vi "Prep_Data_DAQ.vi"(8 "Error  in":errorcluster, 11 "Sequence":T2) -> (0 "Error out":errorcluster, 1 "Time Unit":T1(ring), 2 "Period (s )=Sample Numbers / Sample Frequency":dbl=5.0, 3 "Final Sending Data":u32[](array[numeric]), 4 "Sample Numbers":u32=20000000, 6 "Sample Frequency (Hz)":u32=1000000)   [LabVIEW 2021]
uses:
  DAQ_Control_1.ctl
  Global_DAQ.vi
  <vilib>/Utility/error.llb/Error Cluster From Error Code.vi
  <vilib>/ErrorRing/Error Ring.xnode
panel:
  out "Single line Data":u32[](array[numeric])
  out "Longest length":u32
  out "Array 2":u32[][](array[numeric])
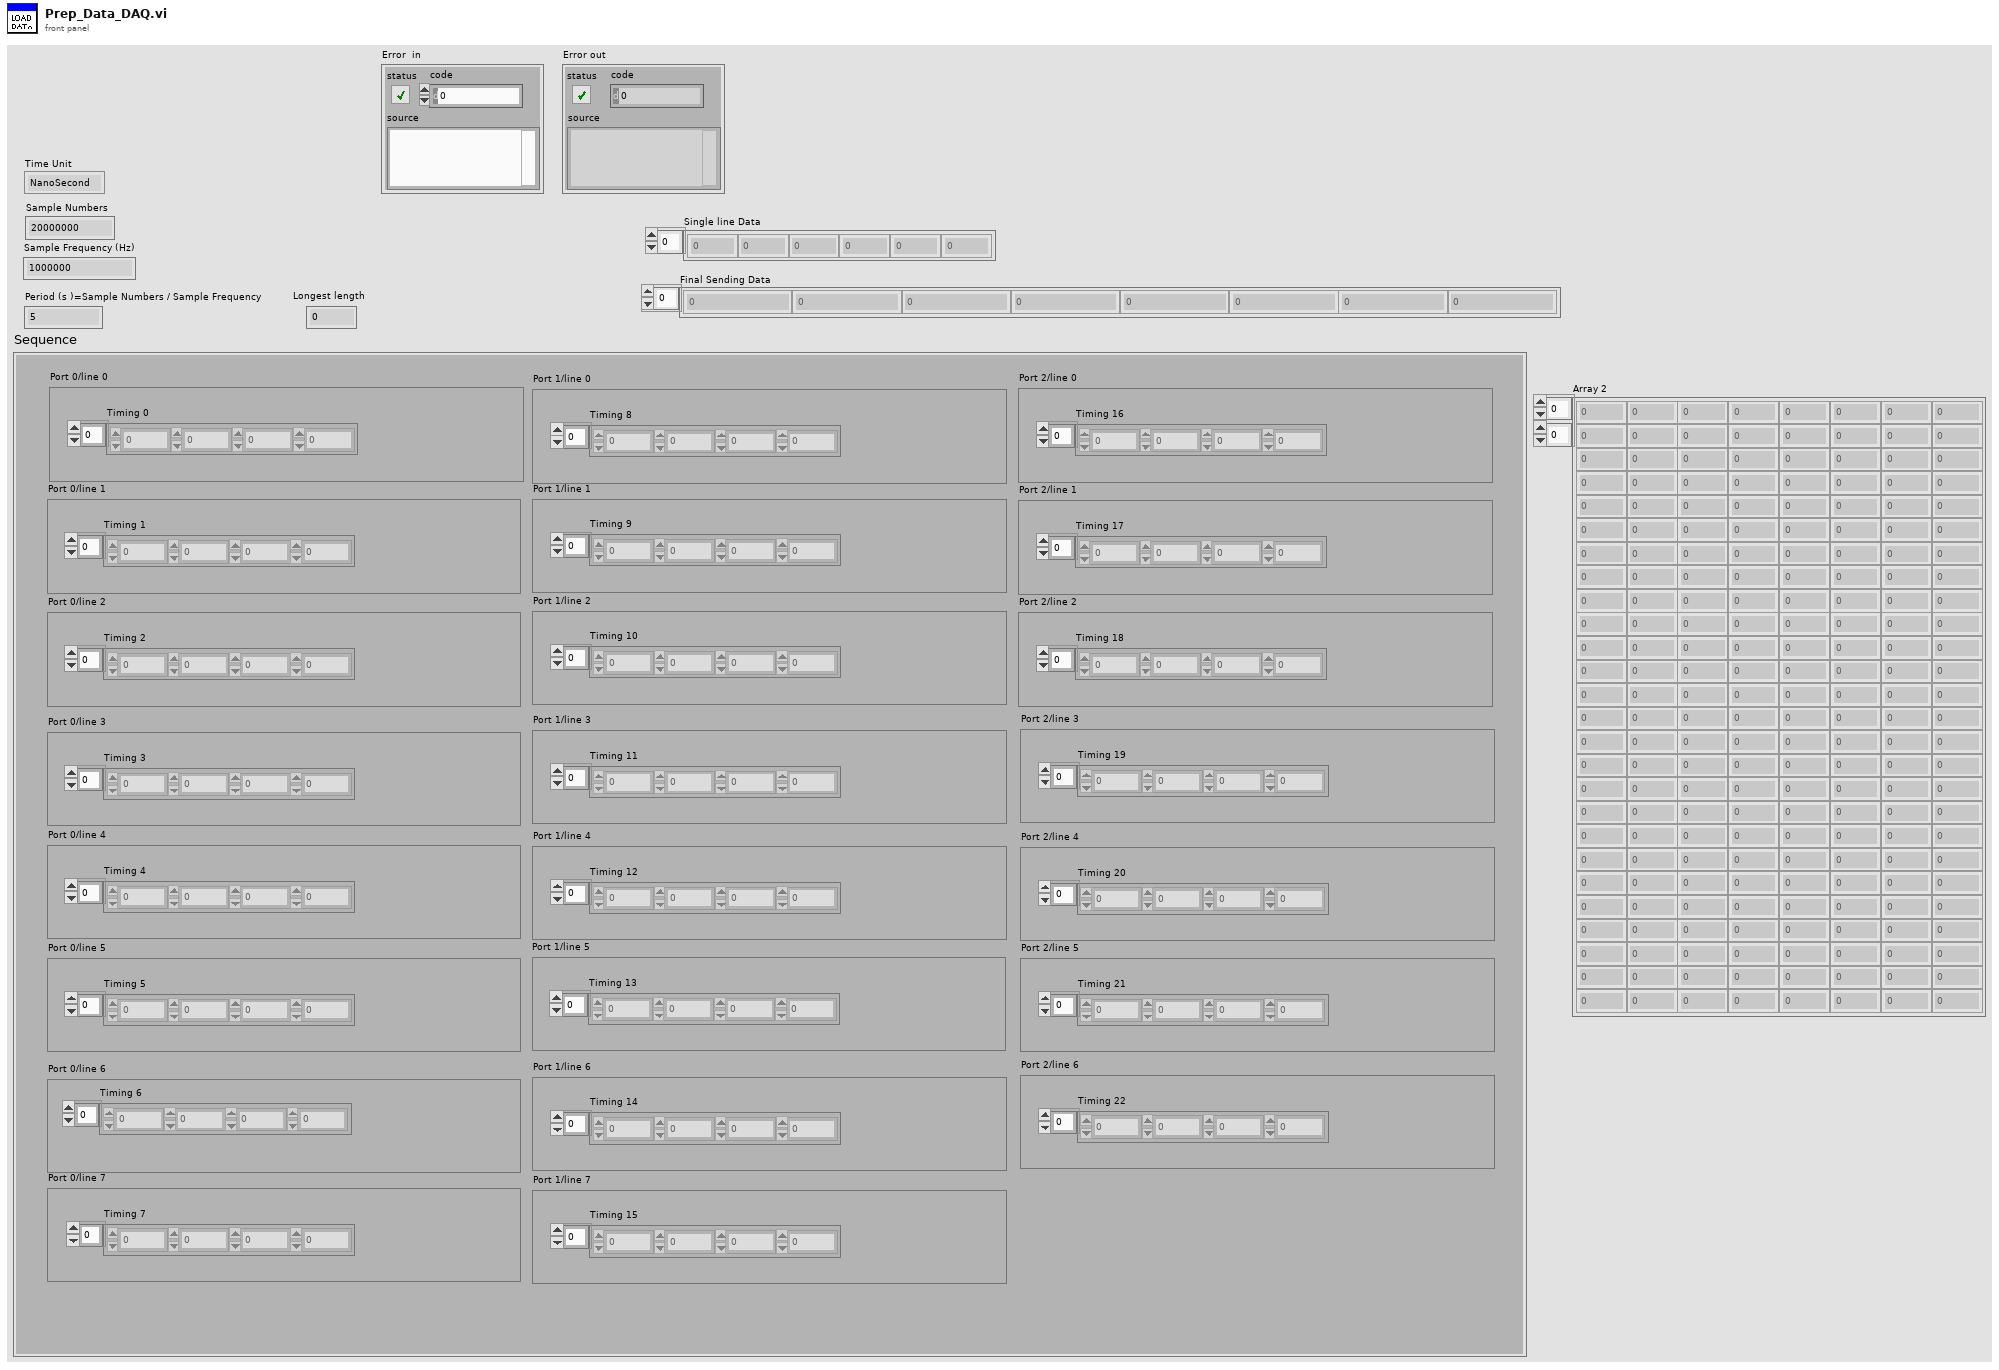
[diagram p1: front panel]
types:
  T1 = enum16{"NanoSecond", "MicroSecond", "MilliSecond"}
  T2 = typedef "DAQ_Control_1.ctl" = cluster{"Port 2/line 6":cluster{"Timing 22":dbl[]}, "Port 2/line 5":cluster{"Timing 21":dbl[]}, "Port 2/line 4":cluster{"Timing 20":dbl[]}, "Port 2/line 3":cluster{"Timing 19":dbl[]}, "Port 2/line 2":cluster{"Timing 18":dbl[]}, "Port 2/line 1":cluster{"Timing 17":dbl[]}, "Port 2/line 0":cluster{"Timing 16":dbl[]}, "Port 1/line 7":cluster{"Timing 15":dbl[]}, "Port 1/line 6":cluster{"Timing 14":dbl[]}, "Port 1/line 5":cluster{"Timing 13":dbl[]}, "Port 1/line 4":cluster{"Timing 12":dbl[]}, "Port 1/line 3":cluster{"Timing 11":dbl[]}, "Port 1/line 2":cluster{"Timing 10":dbl[]}, "Port 1/line 1":cluster{"Timing 9":dbl[]}, "Port 1/line 0":cluster{"Timing 8":dbl[]}, "Port 0/line 7":cluster{"Timing 7\n":dbl[]}, "Port 0/line 6":cluster{"Timing 6\n":dbl[]}, "Port 0/line 5":cluster{"Timing 5\n":dbl[]}, "Port 0/line 4":cluster{"Timing 4\n":dbl[]}, "Port 0/line 3":cluster{"Timing 3\n":dbl[]}, "Port 0/line 2":cluster{"Timing 2":dbl[]}, "Port 0/line 1":cluster{"Timing 1\n":dbl[]}, "Port 0/line 0":cluster{"Timing 0":dbl[]}}
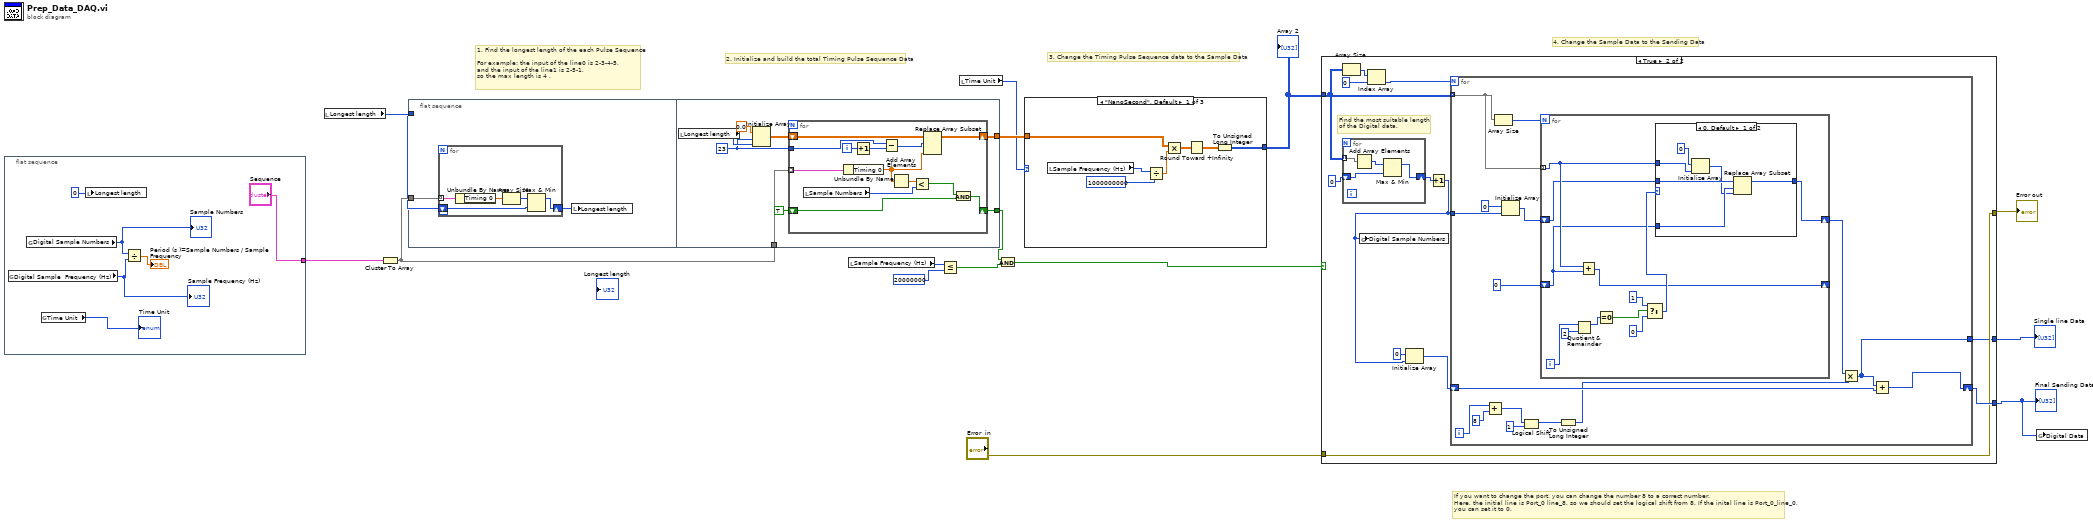
[diagram p0: block diagram]
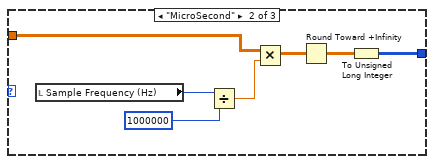
[diagram p2: hidden frame]
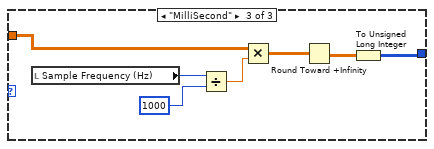
[diagram p3: hidden frame]
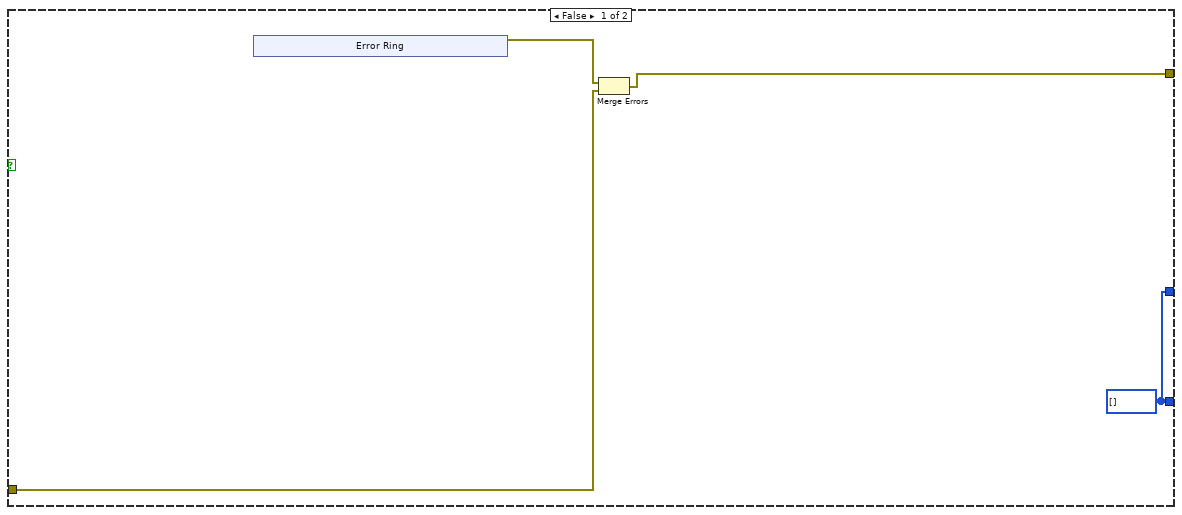
[diagram p4: hidden frame]
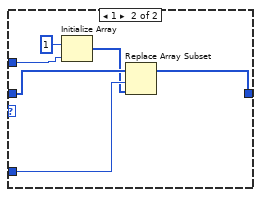
[diagram p5: hidden frame]
diagram:
  # "3. Change the Timing Pulse Sequence data to the Sample Data"
  # "If you want to change the port, you can change the number 8 to a correct number.\nHere, the initial line is Port_0 line_8, so we should set the logical shift from 8. If the inital line is Port_0_line_0, \nyou can set it to 0."
  # "1. Find the longest length of the each Pulse Sequence\n\nFor example: the input of the line0 is 2-3-4-5, \nand the input of the line1 is 2-5-1,\nso the max length is 4 ."
  # "4. Change the Sample Data to the Sending Data"
  # "2. Initialize and build the total Timing Pulse Sequence Data"
  n1 = flat-sequence {
    tunnel: ["Sequence"] -> w4
    frame #0 {
      n2 = global read "Global_DAQ.vi" "Digital Sample  Frequency (Hz)"() -> (w18:u32)
      "Sample Frequency (Hz)" <- w18
      n3 = global read "Global_DAQ.vi" "Digital Sample Numbers"() -> (w19:u32)
      "Sample Numbers" <- w19
      n4 = global read "Global_DAQ.vi" "Time Unit"() -> (→"Time Unit":T1)
      n5 = local write "Longest length"(0) -> ()
      n6 = Divide(x=w19, y=w18) -> (x/y=→"Period (s )=Sample Numbers / Sample Frequency":dbl)
    }
  }
  n7 = local read "Longest length"() -> (w15:u32)
  n8 = Cluster To Array(cluster=w4) -> (array=w14:cluster{"Timing 0":dbl[]}[])
  n9 = flat-sequence {
    tunnel: w15 -> [w22]
    tunnel: w14 -> [w24]
    tunnel: w14 -> [w37]
    tunnel: [w34] -> w3
    tunnel: [w30] -> w8
    frame #0 {
      n10 = for {
        tunnel: w24 -> [w29] mode=indexing
        shift-right: [w26] -> w23
        shift-left: w22 -> [w25]
        n11 = Unbundle By Name(w29) -> ("Timing 0"=w28:dbl[])
        n12 = Array Size(array=w28) -> (size(s)=w27:i32)
        n13 = Max & Min(x=w27, y=w25) -> (max(x,y)=w26:u32)  [unwired: 1 out]
      }
      n14 = local write "Longest length"(w23) -> ()
    }
    frame #1 {
      w32 = 23 ("dimension size")
      n15 = local read "Longest length"() -> (w33:u32)
      n16 = Initialize Array(0.0 ("element"), w32, w33) -> (w35:dbl[][])
      n17 = for {
        tunnel: w37 -> [w50] mode=indexing
        shift-right: [w48] -> w34
        shift-left: w35 -> [w49]
        tunnel: w32 -> [w47]
        shift-right: [w42] -> w30
        shift-left: TRUE -> [w41]
        i -> [w44]
        n18 = local read "Sample Numbers"() -> (w39:u32)
        n19 = Unbundle By Name(w50) -> ("Timing 0"=w43:dbl[])
        n20 = Increment(x=w44) -> (x+1=w45:i32)
        n21 = Subtract(x=w47, y=w45) -> (x-y=w46:i32)
        n22 = Add Array Elements(numeric array=w43) -> (sum=w40:dbl)
        n23 = Less?(x=w40, y=w39) -> (x < y?=w38:bool)
        n24 = Replace Array Subset(array=w49, new element=w43, index (row)=w46) -> (w48:dbl[][])  [unwired: 1 in]
        n25 = And(x=w38, y=w41) -> (x .and. y?=w42:bool)
      }
    }
  }
  n26 = local read "Sample Frequency (Hz)"() -> (w10:u32)
  n27 = Less Or Equal?(x=w10, y=u32 20000000) -> (x <= y?=w7:bool)
  n28 = local read "Time Unit"() -> (w1:T1)
  n29 = And(x=w8, y=w7) -> (x .and. y?=w6:bool)
  n30 = case shown="\"NanoSecond\", Default" w1 {
    tunnel: w3 -> [w57 w64 w70]
    tunnel: [w52 w59 w66] -> w2
    frame "NanoSecond", Default {
      n31 = local read "Sample Frequency (Hz)"() -> (w51:u32)
      n32 = Divide(x=w51, y=u32 1000000000) -> (x/y=w55:dbl)
      n33 = Multiply(x=w57, y=w55) -> (x*y=w54:dbl[][])
      n34 = Round Toward +Infinity(x=w54) -> (ceil(x): smallest int >= x=w53:dbl[][])
      n35 = To Unsigned Long Integer(number=w53) -> (unsigned 32bit integer=w52:u32[][])
    }
    frame "MicroSecond" {
      n36 = local read "Sample Frequency (Hz)"() -> (w58:u32)
      n37 = Divide(x=w58, y=u32 1000000) -> (x/y=w62:dbl)
      n38 = Multiply(x=w64, y=w62) -> (x*y=w61:dbl[][])
      n39 = Round Toward +Infinity(x=w61) -> (ceil(x): smallest int >= x=w60:dbl[][])
      n40 = To Unsigned Long Integer(number=w60) -> (unsigned 32bit integer=w59:u32[][])
    }
    frame "MilliSecond" {
      n41 = local read "Sample Frequency (Hz)"() -> (w65:u32)
      n42 = Divide(x=w65, y=u32 1000) -> (x/y=w71:dbl)
      n43 = Multiply(x=w70, y=w71) -> (x*y=w68:dbl[][])
      n44 = Round Toward +Infinity(x=w68) -> (ceil(x): smallest int >= x=w67:dbl[][])
      n45 = To Unsigned Long Integer(number=w67) -> (unsigned 32bit integer=w66:u32[][])
    }
  }
  "Array 2" <- w2
  n46 = case shown="True" w6 {
    tunnel: w2 -> [_ w84]
    tunnel: [w73 w89] -> w5
    tunnel: "Error  in" -> [w75 w86]
    tunnel: [w74 w86] -> w13
    tunnel: [w73 w85] -> w12
    frame False {
      w73 = u32[] []
      n47 = xnode "Error Ring"() -> ("error out"=w72:errorcluster)
      n48 = Merge Errors(w72, w75) -> (w74:errorcluster)
    }
    frame True {
      # "Find the most suitable length \nof the Digital data."
      n49 = Array Size(array=w84) -> (size(s)=w90:i32[])
      n50 = for {
        tunnel: w84 -> [w96] mode=indexing
        shift-right: [w93] -> w82
        shift-left: 0 -> [w94]
        n51 = Add Array Elements(numeric array=w96) -> (sum=w95:u32)
        n52 = Max & Min(x=w95, y=w94) -> (max(x,y)=w93:u32)  [unwired: 1 out]
      }
      n53 = Index Array(array=w90, index=0) -> (element=w91:i32)
      n54 = Increment(x=w82) -> (x+1=w81:u32)
      n55 = global write "Global_DAQ.vi" "Digital Sample Numbers"(w81) -> ()
      n56 = Initialize Array(u32 0 ("element"), w81) -> (w87:u32[])
      n57 = for {
        N: w91 -> [_]
        tunnel: w84 -> [w112] mode=indexing
        shift-right: [w105] -> w89
        shift-left: w87 -> [w104]
        tunnel: w81 -> [w107]
        tunnel: [w99] -> w85
        i -> [w102]
        n58 = Add(x=w102, y=u32 8) -> (x+y=w100:u32)
        n59 = Array Size(array=w112) -> (size(s)=w108:i32)
        n60 = Initialize Array(u32 0 ("element"), w107) -> (w110:u32[])
        n61 = Logical Shift(y=w100, x=u32 1 ("y")) -> (x << y=w98:u32)
        n62 = for {
          N: w108 -> [_]
          tunnel: w112 -> [w117] mode=indexing
          shift-right: [w116] -> _
          shift-left: u32 0 ("element") -> [w115]
          shift-right: [w113] -> w106
          shift-left: w110 -> [w114]
          i -> [w122]
          n63 = Quotient & Remainder(x=w122, y=2) -> (x-y*floor(x/y)=w120:i32)  [unwired: 1 out]
          n64 = Add(x=w117, y=w115) -> (x+y=w116:u32)
          n65 = Equal To 0?(x=w120) -> (x = 0?=w119:bool)
          n66 = Select(t=u32 1, s=w119, f=u32 0) -> (s? t:f=w118:u32)
          n67 = case shown="0, Default" w118 {
            tunnel: w117 -> [w129 w135]
            tunnel: w114 -> [w127 w134]
            tunnel: w115 -> [w128 w133]
            tunnel: [w125 w131] -> w113
            frame 0, Default {
              n68 = Initialize Array(u32 0 ("element"), w129) -> (w126:u32[])
              n69 = Replace Array Subset(array=w127, new element=w126, index=w128) -> (w125:u32[])
            }
            frame 1 {
              n70 = Initialize Array(u32 1 ("element"), w135) -> (w132:u32[])
              n71 = Replace Array Subset(array=w134, new element=w132, index=w133) -> (w131:u32[])
            }
          }
        }
        n72 = To Unsigned Long Integer(number=w98) -> (unsigned 32bit integer=w97:u32)
        n73 = Multiply(x=w106, y=w97) -> (x*y=w99:u32[])
        n74 = Add(x=w99, y=w104) -> (x+y=w105:u32[])
      }
    }
  }
  "Final Sending Data" <- w5
  "Error out" <- w13
  "Single line Data" <- w12
  n75 = global write "Global_DAQ.vi" "Digital Data"(w5) -> ()
